vi "generator_config.vi"(8 "error in (no error)":errorcluster, 10 "Kalibracni bod":T1, 11 "VISA Refnum in":refnum<visa-resource-name>) -> (0 "error out":errorcluster, 3 "VISA Refnum out":refnum<visa-resource-name>)   [LabVIEW 2022 SP3]
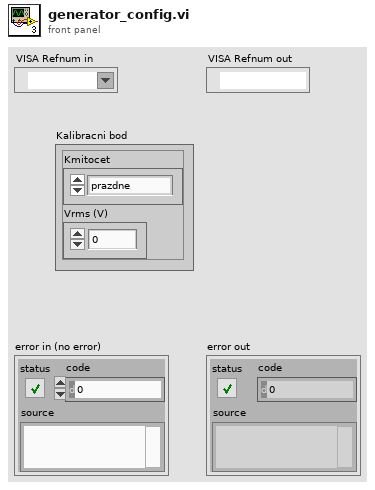
[diagram p1: front panel]
types:
  T1 = cluster{"Kmitocet":enum16{"prazdne", "50 Hz", "1 kHz", "5 kHz", "10 kHz", "20 kHz", "50 kHz", "100 kHz"}, "Vrms (V)":dbl}
  T2 = enum16{"prazdne", "50 Hz", "1 kHz", "5 kHz", "10 kHz", "20 kHz", "50 kHz", "100 kHz"}
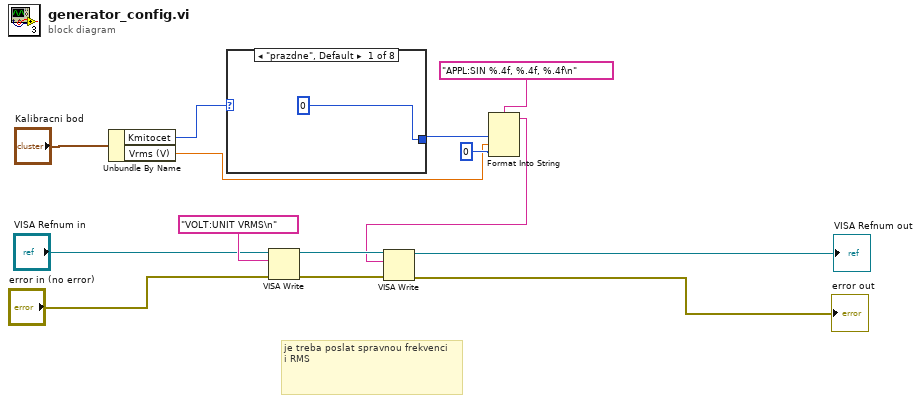
[diagram p0: block diagram]
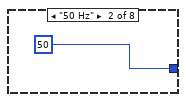
[diagram p2: hidden frame]
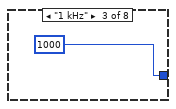
[diagram p3: hidden frame]
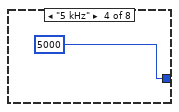
[diagram p4: hidden frame]
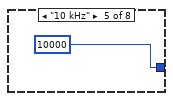
[diagram p5: hidden frame]
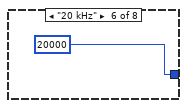
[diagram p6: hidden frame]
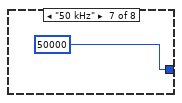
[diagram p7: hidden frame]
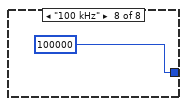
[diagram p8: hidden frame]
diagram:
  # "je treba poslat spravnou frekvenci\ni RMS"
  n1 = Unbundle By Name("Kalibracni bod") -> ("Kmitocet"=w7:T2, "Vrms (V)"=w2:dbl)
  n2 = case shown="\"prazdne\", Default" w7 {
    tunnel: [0 50 1000 5000 10000 20000 50000 100000] -> w5
    frame "prazdne", Default {
    }
    frame "50 Hz" {
    }
    frame "1 kHz" {
    }
    frame "5 kHz" {
    }
    frame "10 kHz" {
    }
    frame "20 kHz" {
    }
    frame "50 kHz" {
    }
    frame "100 kHz" {
    }
  }
  n3 = VISA Write(VISA resource name="VISA Refnum in", write buffer="VOLT:UNIT VRMS\n", error in (no error)="error in (no error)") -> (VISA resource name out=w13:refnum<visa-resource-name>, error out=w14:errorcluster)  [unwired: 1 out]
  n4 = Format Into String(format string="APPL:SIN %.4f, %.4f, %.4f\n" ("write buffer"), w5, w2, 0 ("input 3")) -> (resulting string=w1:string)  [unwired: 2 in, 1 out]
  n5 = VISA Write(VISA resource name=w13, write buffer=w1, error in (no error)=w14) -> (VISA resource name out=→"VISA Refnum out":refnum<visa-resource-name>, error out=→"error out":errorcluster)  [unwired: 1 out]
